vi "Write Parameters to Server.vi"(8 "error out 2":errorcluster, 10 "Experiment Parameter Values":T1(array[cluster]), 11 "connection ID 2":refnum<k5>) -> (0 "error out":errorcluster, 1 "Parameters Set!":bool, 2 "String":string, 3 "connection ID":refnum<k5>)   [LabVIEW 2010, in "Core SubVIs.lvlib"]
uses:
  Core SubVIs.lvlib
panel:
  out "bytes written 3":i32
  out "bytes written 2":i32
  out "bytes written":i32
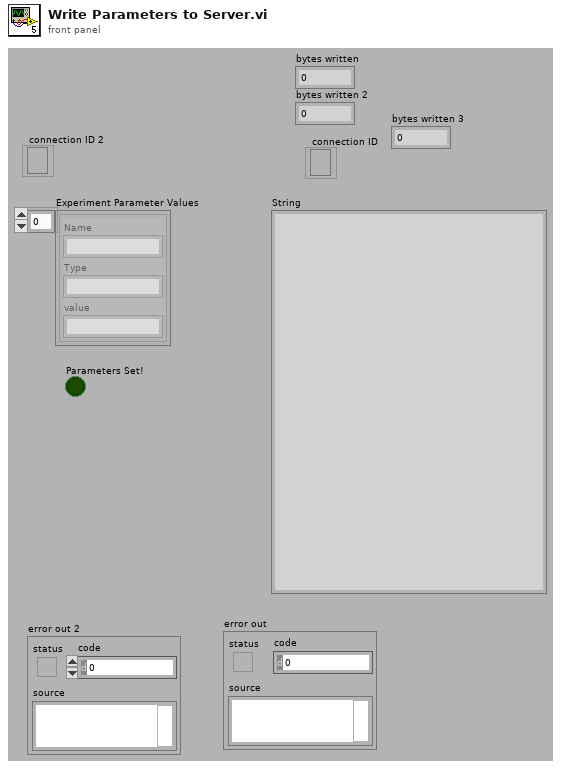
[diagram p1: front panel]
types:
  T1 = cluster{"Name":string, "Type":string, "value":string}[]
  T2 = enum16{"Standard", "Buffered", "CRLF", "Immediate"}
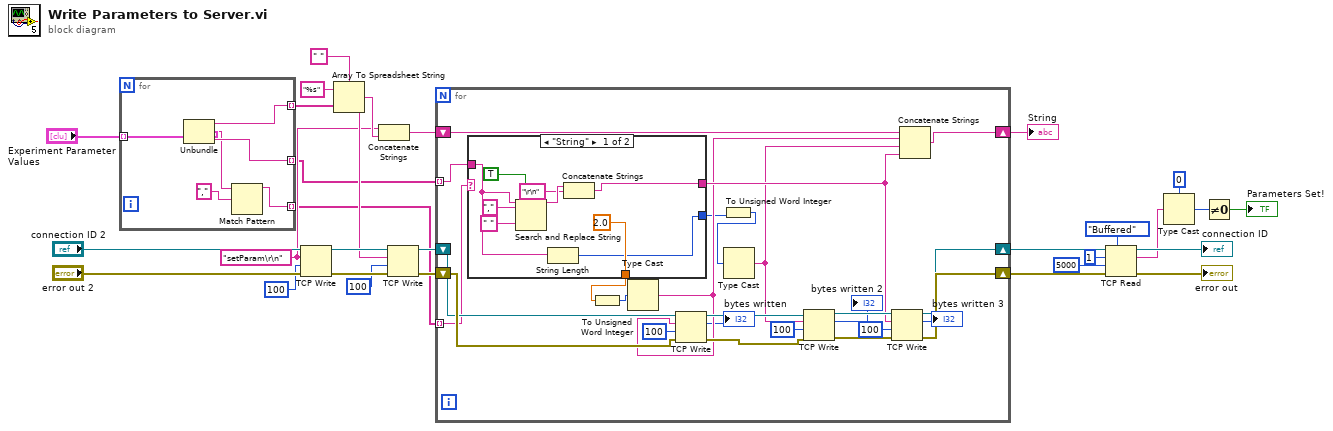
[diagram p0: block diagram]
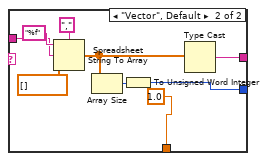
[diagram p2: hidden frame]
diagram:
  w17 = "setParam\r\n" ("data in")
  n1 = for {
    tunnel: [w34] -> w29 mode=indexing
    tunnel: "Experiment Parameter Values" -> [w35] mode=indexing
    tunnel: [w33] -> w3 mode=indexing
    tunnel: [w30] -> w1 mode=indexing
    n2 = Unbundle(w35) -> ("Name"=w34:string, "Type"=w32:string, "value"=w33:string)
    n3 = Match Pattern(string=w32, regular expression=",") -> (before substring=w30:string)  [unwired: 1 in, 3 out]
  }
  n4 = TCP Write(connection ID="connection ID 2", data in=w17, error in (no error)="error out 2", 9:100 ("timeout ms (25000)")) -> (connection ID out=w25:refnum<k5>, error out=w26:errorcluster)  [unwired: 1 out]
  n5 = Array To Spreadsheet String(delimiter (Tab)=" ", array=w29, 3:"%s" ("format string")) -> (spreadsheet string=w18:string)
  n6 = Concatenate Strings(w17, w18) -> (w16:string)
  n7 = TCP Write(connection ID=w25, data in=w18, error in (no error)=w26, 9:100 ("timeout ms (25000)")) -> (connection ID out=w22:refnum<k5>, error out=w21:errorcluster)  [unwired: 1 out]
  n8 = for {
    shift-right: [w59] -> w14
    shift-left: w22 -> [w48]
    shift-right: [w60] -> w13
    shift-left: w21 -> [w51]
    shift-right: [w54] -> w15
    shift-left: w16 -> [w53]
    tunnel: w3 -> [w45] mode=indexing
    tunnel: w1 -> [w46] mode=indexing
    n9 = case shown="\"String\"" w46 {
      tunnel: w45 -> [w61 w74]
      tunnel: [2.0 1.0] -> w44
      tunnel: [w68 w72] -> w38
      tunnel: [w62 w70] -> w43
      frame "String" {
        n10 = Search and Replace String(replace all?=TRUE ("replace all? (F)"), input string=w61, search string=",", replace string=" " ("replace string (\"\")")) -> (result string=w64:string)  [unwired: 4 in, 3 out]
        n11 = String Length(string=w61) -> (length=w68:i32)
        n12 = Concatenate Strings(w64, "\r\n" ("string")) -> (w62:string)
      }
      frame "Vector", Default {
        n13 = Spreadsheet String To Array(delimiter (Tab)=",", format string="%f", spreadsheet string=w74, array type (2D Dbl)=dbl[] []) -> (array=w71:dbl[])
        n14 = Array Size(array=w71) -> (size(s)=w78:i32)
        n15 = To Unsigned Word Integer(number=w78) -> (unsigned 16bit integer=w72:u16)
        n16 = Type Cast(x=w71) -> (*(type *) &x=w70:string)  [unwired: 1 in]
      }
    }
    n17 = To Unsigned Word Integer(number=w44) -> (unsigned 16bit integer=w47:u16)
    n18 = Type Cast(x=w47) -> (*(type *) &x=w41:string)  [unwired: 1 in]
    n19 = TCP Write(connection ID=w48, data in=w41, error in (no error)=w51, 9:100 ("timeout ms (25000)")) -> (connection ID out=w49:refnum<k5>, bytes written=→"bytes written":i32, error out=w50:errorcluster)
    n20 = To Unsigned Word Integer(number=w38) -> (unsigned 16bit integer=w37:u16)
    n21 = Type Cast(x=w37) -> (*(type *) &x=w42:string)  [unwired: 1 in]
    n22 = TCP Write(connection ID=w49, data in=w42, error in (no error)=w50, 9:100 ("timeout ms (25000)")) -> (connection ID out=w56:refnum<k5>, bytes written=→"bytes written 2":i32, error out=w55:errorcluster)
    n23 = TCP Write(connection ID=w56, data in=w43, error in (no error)=w55, 9:100 ("timeout ms (25000)")) -> (connection ID out=w59:refnum<k5>, bytes written=→"bytes written 3":i32, error out=w60:errorcluster)
    n24 = Concatenate Strings(w53, w41, w42, w43) -> (w54:string)
  }
  "String" <- w15
  n25 = TCP Read(connection ID=w14, bytes to read=1, error in (no error)=w13, 7:T2."Buffered" ("mode (standard)"), 9:5000 ("timeout ms (25000)")) -> (connection ID out=→"connection ID":refnum<k5>, data out=w5:string, error out=→"error out":errorcluster)
  n26 = Type Cast(type=u8 0, x=w5) -> (*(type *) &x=w6:u8)
  n27 = Not Equal To 0?(x=w6) -> (x != 0?=→"Parameters Set!":bool)
